vi "Init.vi"(8 "error in (no error)":errorcluster) -> (0 "error out":errorcluster, 3 "reference out":refnum<k24>)   [LabVIEW 2019, in "LabNation Scope Driver.lvlib"]
doc: "Initializes the Smart Scope."
uses:
  LabNation Scope Driver.lvlib
  C:/Program Files (x86)/LabNation/SmartScope/DeviceInterface.dll
  Program Files (x86)/LabNation/SmartScope/DeviceInterface.dll
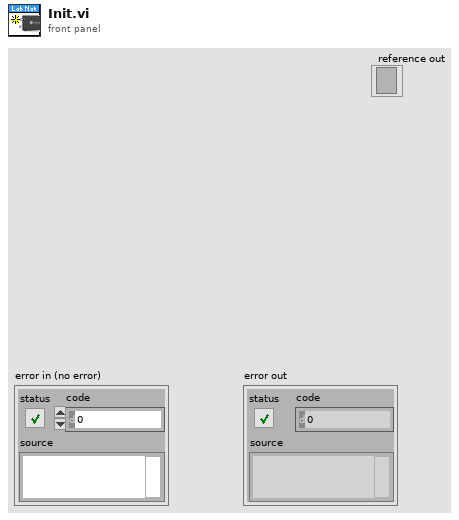
[diagram p1: front panel]
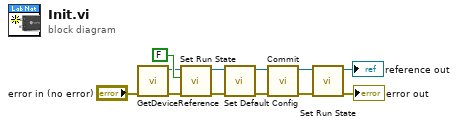
[diagram p0: block diagram]
diagram:
  n1 = call "GetDeviceReference.vi"("error in (no error)"="error in (no error)") -> ("error out"=w10:errorcluster, "MainDevice Reference"=w11:refnum<k24>)  [unwired: 9 in]
  n2 = call "Set Run State.vi"("error in (no error)"=w10, "RunState(T)"=FALSE ("RunState"), "reference in"=w11) -> ("error out"=w8:errorcluster, "reference out"=w9:refnum<k24>)  [unwired: 7 in]
  n3 = call "Set Default Config.vi"("error in (no error)"=w8, "reference in"=w9) -> ("error out"=w6:errorcluster, "reference out"=w7:refnum<k24>)  [unwired: 8 in]
  n4 = call "Commit.vi"("error in (no error)"=w6, "reference in"=w7) -> ("error out"=w5:errorcluster, "reference out"=w4:refnum<k24>)  [unwired: 8 in]
  n5 = call "Set Run State.vi"("error in (no error)"=w5, "reference in"=w4) -> ("error out"=→"error out":errorcluster, "reference out"=→"reference out":refnum<k24>)  [unwired: 8 in]
